vi "Configuration 1.2 JSON Unflatten.vi"(8 "error in (no error)":errorcluster, 11 "dsf configuration json":string) -> (0 "error out":errorcluster, 3 "configuration 1.2":T1={"plugins"=[{"name"="", "components"=[], "cycle timing"={"priority"=100, "decimation"=1, "offset"=0}, "threads"=[{"processor"=-2, "priority offset"=0, "settings"=[]}, {"processor"=-2, "priority offset"=0, "settings"=[]}, {"processor"=-2, "priority offset"=0, "settings"=[]}, {"processor"=-2, "priority offset"=0, "settings"=[]}], "transfer groups"=[{"name"="", "direction"=enum."Tx", "cycle timing"={"priority"=100, "decimation"=1, "offset"=0}, "thread index"=0, "settings"=[], "transfers"=[{"name"="", "byte order"=enum."big-endian", "settings"=[], "channels"=[]}], "timeout behavior"=enum."Increment Late Count"}], "settings"=[]}]})   [LabVIEW 2017, in "DSF Core.lvlib" / "Configuration Session.lvclass"]
uses:
  Configuration Session.lvclass
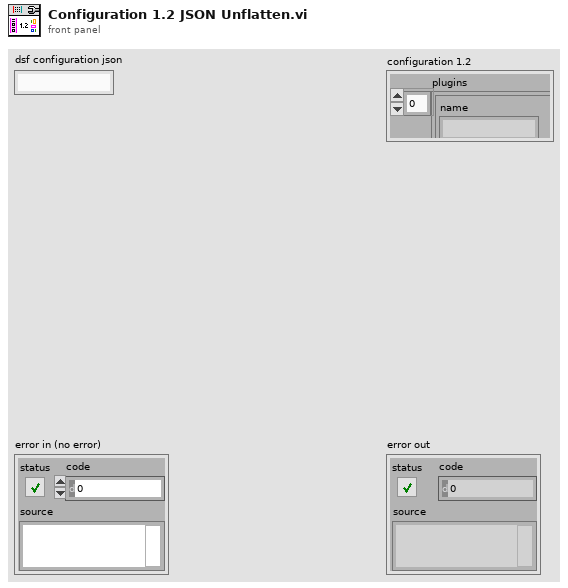
[diagram p1: front panel]
types:
  T1 = cluster{"plugins":cluster{"name":string, "components":string[], "cycle timing":cluster{"priority":u64, "decimation":u64, "offset":u64}, "threads":cluster{"processor":i32, "priority offset":i16, "settings":cluster{"component":string, "name":string, "values":cluster{"key":string, "value":string}[]}[]}[], "transfer groups":cluster{"name":string, "direction":enum8{"Tx", "Rx"}, "cycle timing":cluster{"priority":u64, "decimation":u64, "offset":u64}, "thread index":i32, "settings":cluster{"component":string, "name":string, "values":cluster{"key":string, "value":string}[]}[], "transfers":cluster{"name":string, "byte order":enum8{"big-endian", "little-endian"}, "settings":cluster{"component":string, "name":string, "values":cluster{"key":string, "value":string}[]}[], "channels":cluster{"string offset":u64, "name":string, "units":string, "engine data type":enum8{"Bool", "SGL", "DBL", "I8", "I16", "I32", "I64", "U8", "U16", "U32", "U64"}, "string data type":enum8{"Bool", "SGL", "DBL", "I8", "I16", "I32", "I64", "U8", "U16", "U32", "U64"}, "settings":cluster{"component":string, "name":string, "values":cluster{"key":string, "value":string}[]}[]}[]}[], "timeout behavior":enum8{"Increment Late Count", "Throw Error"}}[], "settings":cluster{"component":string, "name":string, "values":cluster{"key":string, "value":string}[]}[]}[]}
  T2 = cluster{"plugins":cluster{"name":string, "components":string[], "cycle timing":cluster{"priority":u64, "decimation":u64, "offset":u64}, "threads":cluster{"processor":i32, "priority offset":i16, "settings":cluster{"component":string, "name":string, "values":cluster{"key":string, "value":string}[]}[]}[], "transfer groups":cluster{"name":string, "direction":u8, "cycle timing":cluster{"priority":u64, "decimation":u64, "offset":u64}, "thread index":i32, "settings":cluster{"component":string, "name":string, "values":cluster{"key":string, "value":string}[]}[], "transfers":cluster{"name":string, "byte order":u8, "settings":cluster{"component":string, "name":string, "values":cluster{"key":string, "value":string}[]}[], "channels":cluster{"string offset":u64, "name":string, "units":string, "engine data type":u8, "string data type":u8, "settings":cluster{"component":string, "name":string, "values":cluster{"key":string, "value":string}[]}[]}[]}[], "timeout behavior":u8}[], "settings":cluster{"component":string, "name":string, "values":cluster{"key":string, "value":string}[]}[]}[]}
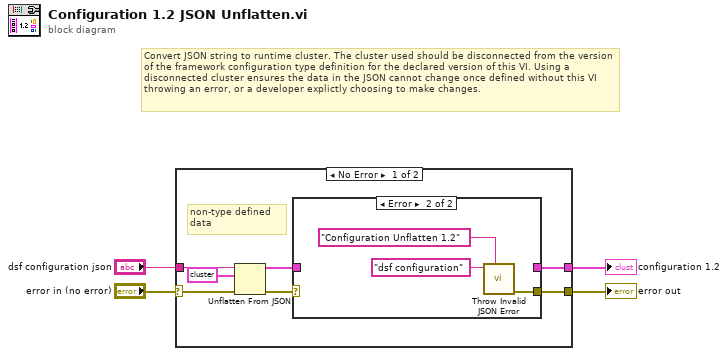
[diagram p0: block diagram]
diagram:
  # "Convert JSON string to runtime cluster. The cluster used should be disconnected from the version of the framework configuration type definition for the declared version of this VI. Using a disconnected cluster ensures the data in the JSON cannot change once defined without this VI throwing an error, or a developer explictly choosing to make changes."
  n1 = case shown="No Error" "error in (no error)" {
    selector: "error in (no error)" -> [w6 w17]
    tunnel: "dsf configuration json" -> [w11 _]
    tunnel: [w9 w17] -> w3
    tunnel: [w7 _] -> w1
    frame No Error {
      # "non-type defined data"
      n2 = Unflatten From JSON(JSON string=w11, type and defaults=T2 {"plugins"=[{"name"="", "components"=[], "cycle timing"={"priority"=100, "decimation"=1, "offset"=0}, "threads"=[{"processor"=-2, "priority offset"=0, "settings"=[]}, {"processor"=-2, "priority offset"=0, "settings"=[]}, {"processor"=-2, "priority offset"=0, "settings"=[]}, {"processor"=-2, "priority offset"=0, "settings"=[]}], "transfer groups"=[{"name"="", "direction"=0, "cycle timing"={"priority"=100, "decimation"=1, "offset"=0}, "thread index"=0, "settings"=[], "transfers"=[{"name"="", "byte order"=0, "settings"=[], "channels"=[]}], "timeout behavior"=0}], "settings"=[]}]} ("framework configuration 1.2"), error in (no error)=w6) -> (value=w8:T2, error out=w10:errorcluster)  [unwired: 4 in]
      n3 = case shown="Error" w10 {
        selector: w10 -> [w13 _]
        tunnel: [w13 w16] -> w9
        tunnel: w8 -> [w12 _]
        tunnel: [w12 _] -> w7
        frame No Error {
        }
        frame Error {
          n4 = call "Throw Invalid JSON Error.vi"("error source vi name"="Configuration Unflatten 1.2", "name"="dsf configuration") -> ("error out"=w16:errorcluster)  [unwired: 9 in]
        }
      }
    }
    frame Error {
    }
  }
  "error out" <- w3
  "configuration 1.2" <- w1
